vi "WMI Serial Query.vi"(8 "error in":errorcluster) -> (0 "error out":errorcluster, 2 "Description":string[](array[string]), 3 "MAC Addresses":string[](array[string]))   [LabVIEW 2012]
uses:
  System.Management
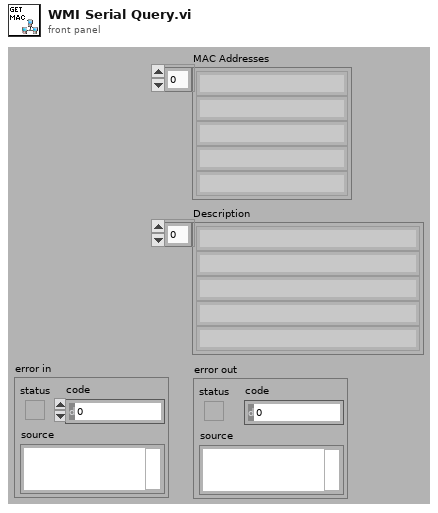
[diagram p1: front panel]
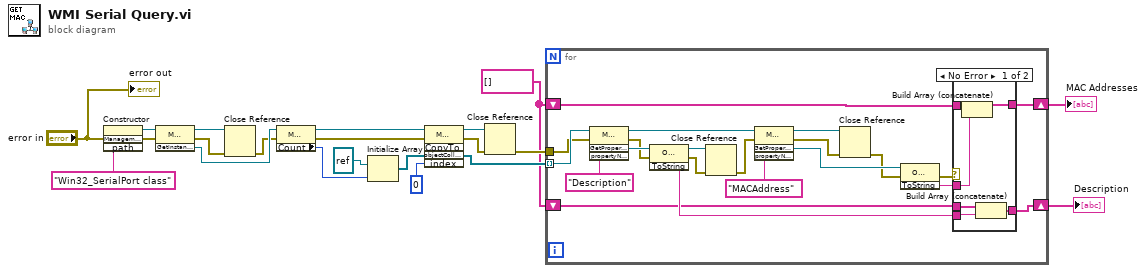
[diagram p0: block diagram]
diagram:
  w1 = string[] []
  n1 = constructor class="ManagementClass"(error in="error in", "path"="Win32_SerialPort class") -> (reference out=w20:refnum<k24>, error out=w13:errorcluster)  [unwired: 2 in, 2 out]
  n2 = invoke class="ManagementClass" method="GetInstances"(reference=w20, error in=w13) -> (reference out=w6:refnum<k24>, error out=w5:errorcluster, "GetInstances"=w18:refnum<k24>)  [unwired: 1 in]
  n3 = Close Reference(reference=w6, error in (no error)=w5) -> (error out=w4:errorcluster)
  n4 = property class="ManagementObjectCollection"(reference=w18, error in=w4) -> (reference out=w11:refnum<k24>, error out=w10:errorcluster, "Count"=w17:i32)
  n5 = Initialize Array(refnum<k24> refnum, w17) -> (w16:refnum<k24>[])
  n6 = invoke on="Invoke Node" class="ManagementObjectCollection" method="CopyTo"(reference=w11, error in=w10, "objectCollection"=w16, "index"=0) -> (reference out=w9:refnum<k24>, error out=w8:errorcluster, "objectCollection"=w14:refnum<k24>[])  [unwired: 1 in, 2 out]
  n7 = Close Reference(reference=w9, error in (no error)=w8) -> (error out=w7:errorcluster)
  n8 = for {
    tunnel: w14 -> [w42] mode=indexing
    shift-right: [w39] -> w12
    shift-left: w1 -> [w38]
    tunnel: w7 -> [w37]
    shift-right: [w23] -> w3
    shift-left: w1 -> [w24]
    n9 = invoke class="ManagementBaseObject" method="GetPropertyValue"(reference=w42, error in=w37, "propertyName"="Description") -> (reference out=w35:refnum<k24>, error out=w36:errorcluster, "GetPropertyValue"=w40:refnum<k24>)  [unwired: 1 in, 1 out]
    n10 = invoke class="Object" method="ToString"(reference=w40, error in=w36) -> (reference out=w34:refnum<k24>, error out=w33:errorcluster, "ToString"=w28:string)  [unwired: 1 in]
    n11 = Close Reference(reference=w34, error in (no error)=w33) -> (error out=w32:errorcluster)
    n12 = invoke class="ManagementBaseObject" method="GetPropertyValue"(reference=w35, error in=w32, "propertyName"="MACAddress") -> (reference out=w31:refnum<k24>, error out=w27:errorcluster, "GetPropertyValue"=w30:refnum<k24>)  [unwired: 1 in, 1 out]
    n13 = Close Reference(reference=w31, error in (no error)=w27) -> (error out=w26:errorcluster)
    n14 = invoke class="Object" method="ToString"(reference=w30, error in=w26) -> (error out=w25:errorcluster, "ToString"=w29:string)  [unwired: 1 in, 1 out]
    n15 = case shown="No Error" w25 {
      tunnel: [w48 w50] -> w39
      tunnel: w38 -> [w47 w50]
      tunnel: w29 -> [w46 _]
      tunnel: w28 -> [w44 _]
      tunnel: w24 -> [w45 w49]
      tunnel: [w43 w49] -> w23
      frame No Error {
        n16 = Build Array (concatenate)(w47, w46) -> (w48:string[])
        n17 = Build Array (concatenate)(w45, w44) -> (w43:string[])
      }
      frame Error {
      }
    }
  }
  "MAC Addresses" <- w12
  "Description" <- w3
  "error out" <- "error in"
